vi "TurnToAngle.vi"(10 "AllowedDeviation":dbl=2.4 format="%#_13g", 11 "GyroValue":dbl) -> ()   [LabVIEW 2015]
uses:
  <vilib>/addons/control/pid/pid.llb/PID (DBL).vi
  <vilib>/addons/control/pid/NI_PID_pid.lvlib
  navx-mxp/labview/navX Library v2/navX Library v2.lvlib
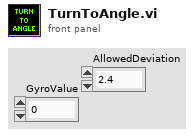
[diagram p1: front panel]
types:
  T1 = typedef "WPI_MotorControlDeviceRef.ctl" = cluster{"DeviceStatus":errorcluster, "Type":T2, "PWM":cluster{"PWM Channel":T3, "DeadBand":T4}, "CAN":cluster{"Device Number":u8, "Control Mode":T5, "Semaphore":T6, "Max Vout":dbl, "TalonSRX Control Mode":T7}, "Invert":bool}
  T2 = typedef "WPI_MotorControlType.ctl" = enum16{"PWM", "CAN", "CANTalonSRX"}
  T3 = typedef "FPGA_DIOPWMChannel.ctl" = enum8{"PWM 0", "PWM 1", "PWM 2", "PWM 3", "PWM 4", "PWM 5", "PWM 6", "PWM 7", "PWM 8", "PWM 9", "PWM MXP 0", "PWM MXP 1", "PWM MXP 2", "PWM MXP 3", "PWM MXP 4", "PWM MXP 5", "PWM MXP 6", "PWM MXP 7", "PWM MXP 8", "PWM MXP 9", "Invalid"}
  T4 = typedef "WPI_PWMDeadband.ctl" = cluster{"Name":string, "maxPositivePwm":i32, "minPositivePwm":i32, "centerPwm":i32, "maxNegativePwm":i32, "minNegativePwm":i32, "angularRange":u16}
  T5 = typedef "WPI_CANJaguar_ControlMode.ctl" = enum8{"Percent VBus", "Current", "Speed", "Position", "Voltage"}
  T6 = typedef "Semaphore RefNum" = refnum<k1>
  T7 = typedef "WPI_CANTalonSRX_APIControlMode.ctl" = enum8{"Percent VBus", "Speed", "Position", "Slave", "Unchanged / Invalid", "Voltage Compensation", "Current", "Motion Profile"}
  T8 = typedef "navX Library v2.lvlib/Z900_navX_DeviceTypeDef.ctl" = cluster{"Interface":cluster{"Protocol":T9, "Update Rate (4Hz-60Hz)":u8, "navX Open TypeDef":variant}, "Notify Packet":refnum<notifier>, "Loop VI Refnum":refnum<vi>, "Ready to Close Occurrence Refnum":refnum<k4>}
  T9 = typedef "navX Library v2.lvlib/Z900_navX_ProtocolTypeDef.ctl" = enum16{"SERIAL", "I2C", "SPI"}
  T10 = cluster{"proportional gain (Kc)":dbl, "integral time (Ti, min)":dbl, "derivative time (Td, min)":dbl}
  T11 = cluster{"Yaw":dbl, "Roll":dbl, "Pitch":dbl, "Heading":dbl, "Fused Heading":dbl}
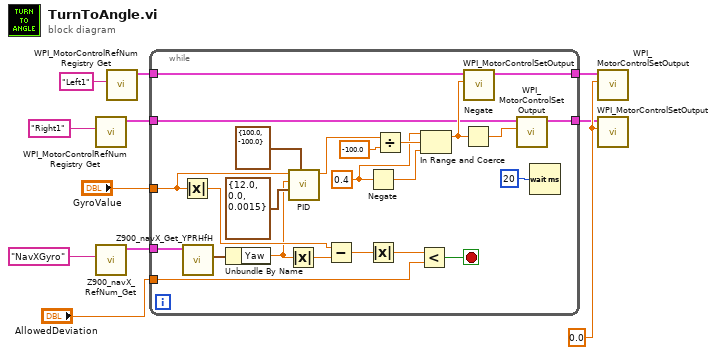
[diagram p0: block diagram]
diagram:
  w10 = 0.0 ("Output")
  n1 = call <vilib>:"WPI_MotorControlRefNum Registry Get.vi"("refnum name"="Right1") -> ("MotorControlDevRef"=w5:T1)  [unwired: 9 in, 1 out]
  n2 = call "Z900_navX_RefNum_Get.vi"("refnum name"="NavXGyro") -> ("navX Device"=w1:T8)  [unwired: 9 in, 1 out]
  n3 = call <vilib>:"WPI_MotorControlRefNum Registry Get.vi"("refnum name"="Left1") -> ("MotorControlDevRef"=w3:T1)  [unwired: 9 in, 1 out]
  n4 = while {
    tunnel: w1 -> [w12]
    tunnel: [w20] -> w8
    tunnel: [w19] -> w9
    tunnel: "GyroValue" -> [w18]
    tunnel: "AllowedDeviation" -> [w17]
    tunnel: w5 -> [w16]
    tunnel: w3 -> [w15]
    stop <- w21 stop-if-true
    w27 = 0.4 ("upper limit")
    n5 = Absolute Value(x=w18) -> (abs(x)=w25:dbl)
    n6 = call "Z900_navX_Get_YPRHfH.vi"("navX Device"=w12) -> ("YRPHfH"=w14:T11)  [unwired: 7 in, 3 out]
    n7 = Unbundle By Name(w14) -> ("Yaw"=w13:dbl)
    n8 = Absolute Value(x=w13) -> (abs(x)=w24:dbl)
    n9 = call-poly <vilib>:"PID.vi"("output range"=cluster{"output high":dbl, "output low":dbl} {"output high"=100.0, "output low"=-100.0}, "PID gains"=T10 {"proportional gain (Kc)"=12.0, "integral time (Ti, min)"=0.0, "derivative time (Td, min)"=0.0015}, "process variable"=w13, "setpoint"=w18) -> ("output"=w30:dbl)  [unwired: 6 in, 1 out]
    n10 = Subtract(x=w25, y=w24) -> (x-y=w23:dbl)
    n11 = Negate(x=w27) -> (-x=w26:dbl)
    n12 = Absolute Value(x=w23) -> (abs(x)=w22:dbl)
    n13 = Divide(x=w30, y=-100.0) -> (x/y=w28:dbl)
    n14 = Less?(x=w22, y=w17) -> (x < y?=w21:bool)
    n15 = In Range and Coerce(upper limit=w27, x=w28, lower limit=w26) -> (coerced(x)=w35:dbl)  [unwired: 1 out]
    n16 = Negate(x=w35) -> (-x=w34:dbl)
    n17 = call <vilib>:"WPI_MotorControlSetOutput.vi"("Output"=w35, "MotorControlDevRef"=w15) -> ("MotorControlDevRef"=w19:T1)  [unwired: 7 in, 2 out]
    n18 = call <vilib>:"WPI_MotorControlSetOutput.vi"("Output"=w34, "MotorControlDevRef"=w16) -> ("MotorControlDevRef"=w20:T1)  [unwired: 7 in, 2 out]
    n19 = Wait (ms)(milliseconds to wait=u32 20) -> ()  [unwired: 1 out]
  }
  n20 = call <vilib>:"WPI_MotorControlSetOutput.vi"("Output"=w10, "MotorControlDevRef"=w9) -> ()  [unwired: 7 in, 3 out]
  n21 = call <vilib>:"WPI_MotorControlSetOutput.vi"("Output"=w10, "MotorControlDevRef"=w8) -> ()  [unwired: 7 in, 3 out]
